vi "Get Calibrated Data per Site.vi"(0 "TSM context":T2, 11 "error in (no error)":errorcluster) -> (4 "Per Site Acoustic Cal Data":T1[](array[typedef]), 6 "Found?":bool, 15 "error out":errorcluster)   [LabVIEW 2020]
doc: "Gets the Acoustic Calibration Data for the all Sites by reading the Site Data from TSM context."
uses:
  <vilib>/NI_TestStand_SemiconductorModule/NI_TestStand_Semiconductor_Module.lvlibp/PinMap/General/SemiconductorModuleContext.ctl
  Common/Utility/Calibration File API/Acoustic Cal Data Cluster.ctl
  <vilib>/NI_TestStand_SemiconductorModule/NI_TestStand_Semiconductor_Module.lvlibp
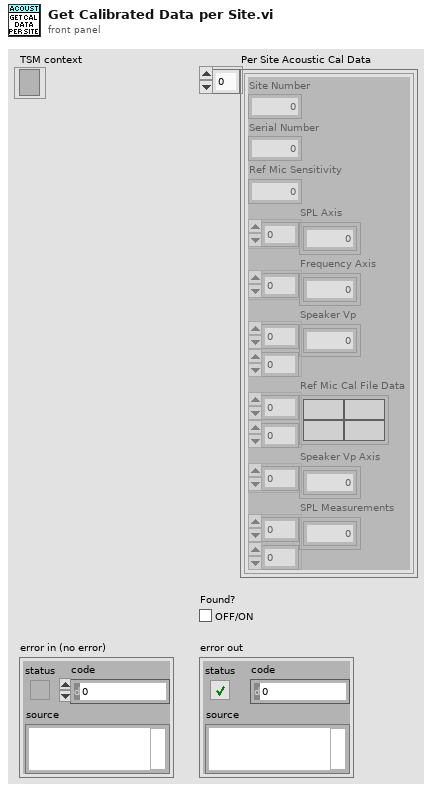
[diagram p1: front panel]
types:
  T1 = typedef "Acoustic Cal Data Cluster.ctl" = cluster{"Site Number":i32, "Serial Number":u32, "Ref Mic Sensitivity":dbl, "SPL Axis":dbl[], "Frequency Axis":dbl[], "Speaker Vp":dbl[][], "Ref Mic Cal File Data":string[][], "Speaker Vp Axis":dbl[], "SPL Measurements":dbl[][]}
  T2 = typedef "NI_TestStand_Semiconductor_Module.lvlibp/SemiconductorModuleContext.ctl" = refnum<k7>
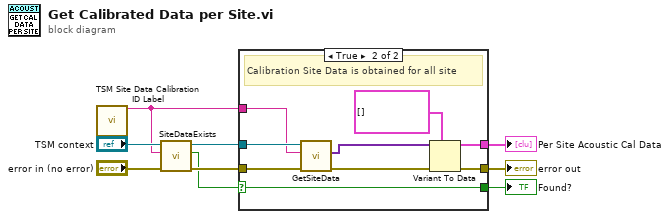
[diagram p0: block diagram]
diagram:
  n1 = call "TSM Site Data Calibration ID Label.vi"() -> ("Calibration Data Id"=w5:string)  [unwired: 15 in]
  n2 = call <vilib>:"SiteDataExists.vi"("error in (no error)"="error in (no error)", "Data Id"=w5, "Semiconductor Module Context"="TSM context") -> ("error out"=w7:errorcluster, "Site Data Exists?"=w2:bool, "Semiconductor Module Context Out"=w6:T2)  [unwired: 6 in]
  n3 = case shown="True" w2 {
    selector: w2 -> [w10 w13]
    tunnel: w7 -> [w11 w20]
    tunnel: w6 -> [_ w19]
    tunnel: w5 -> [_ w18]
    tunnel: [w11 w15] -> w4
    tunnel: [_ w14] -> w1
    tunnel: [w10 w13] -> w3
    frame False {
      # "Not calibration data found"
    }
    frame True {
      # "Calibration Site Data is obtained for all site"
      n4 = call <vilib>:"GetSiteData.vi"("error in (no error)"=w20, "Data Id"=w18, "Semiconductor Module Context"=w19) -> ("error out"=w16:errorcluster, "Site Data"=w17:variant[])  [unwired: 6 in, 1 out]
      n5 = Variant To Data(error in=w16, type=T1[] [], Variant=w17) -> (data=w14:T1[], error out=w15:errorcluster)
    }
  }
  "error out" <- w4
  "Found?" <- w3
  "Per Site Acoustic Cal Data" <- w1
